vi "testPeriodicStateString.vi"(8 "error in (no error)":errorcluster, 11 "testStateMachineUtilities in":refnum<class "testStateMachineUtilities.lvclass">) -> (0 "error out":errorcluster, 3 "testStateMachineUtilities out":refnum<class "testStateMachineUtilities.lvclass">)   [LabVIEW 2013, in "testStateMachineUtilities.lvclass"]
uses:
  testStateMachineUtilities.lvclass
  source/State Machine Support API/Conditional State String.vi
  <userlib>/_OpenG.lib/time/time.llb/Periodic Trigger__ogtk.vi
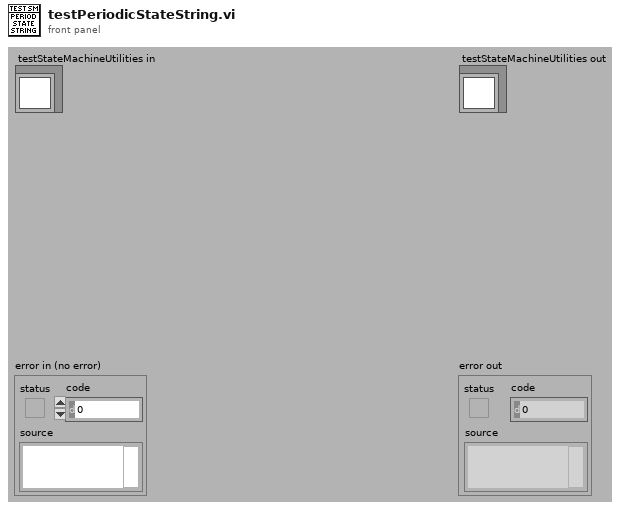
[diagram p1: front panel]
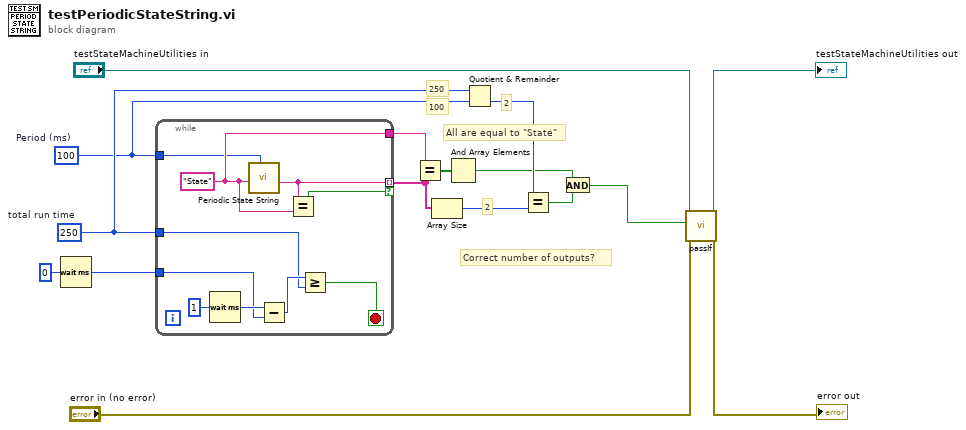
[diagram p0: block diagram]
diagram:
  w6 = u32 100  # Period (ms)
  w7 = u32 250  # total run time
  # "Correct number of outputs?"
  # "2"
  # "2"
  # "100"
  # "250"
  # "All are equal to \"State\""
  n1 = Wait (ms)(milliseconds to wait=u32 0) -> (millisecond timer value=w11:u32)
  n2 = while {
    tunnel: [w26] -> w8 mode=indexing if=w25
    tunnel: w11 -> [w22]
    tunnel: w7 -> [w18]
    tunnel: [w21] -> w10
    tunnel: w6 -> [w20]
    stop <- w17 stop-if-true
    w21 = "State" ("State Queue")
    n3 = Wait (ms)(milliseconds to wait=u32 1) -> (millisecond timer value=w23:u32)
    n4 = call "Periodic State String.vi"("Period (ms)"=w20, "State"=w21) -> ("State Out"=w26:string)  [unwired: 9 in]
    n5 = Subtract(x=w23, y=w22) -> (x-y=w19:u32)
    n6 = Equal?(x=w26, y=w21) -> (x = y?=w25:bool)
    n7 = Greater Or Equal?(x=w19, y=w18) -> (x >= y?=w17:bool)
  }
  n8 = Equal?(x=w10, y=w8) -> (x = y?=w9:bool[])
  n9 = Array Size(array=w8) -> (size(s)=w4:i32)
  n10 = And Array Elements(Boolean array=w9) -> (logical AND=w2:bool)
  n11 = Quotient & Remainder(x=w7, y=w6) -> (floor(x/y)=w5:u32)  [unwired: 1 out]
  n12 = Equal?(x=w5, y=w4) -> (x = y?=w3:bool)
  n13 = And(x=w2, y=w3) -> (x .and. y?=w1:bool)
  n14 = call-dynamic "passIf.vi"("error in (no error)"="error in (no error)", "pass"=w1, "TestCase in"="testStateMachineUtilities in") -> ("error out"=→"error out":errorcluster, "TestCase out"=→"testStateMachineUtilities out":refnum<class "testStateMachineUtilities.lvclass">)  [unwired: 7 in]
